vi "Teleop.vi"(10 "Match Info":T1={"Autonomous Elapsed Seconds"=0.0, "TeleOp Elapsed Seconds"=0.0, "Disabled Elapsed Seconds"=0.0, "Visited Autonomous"=FALSE, "Visited TeleOp"=FALSE, "Visited Disabled"=FALSE, "Autonomous Settings"={"Autonomous Style"=enum."Independent", "VI Refnum"=refnum}}, 11 "Call Context":T2) -> ()   [LabVIEW 2015]
doc: "This VI is called for each TeleOp packet received from the DS where the robot is not disabled. It is often used to read from the joysticks and update I/O or to update setpoints for timed control loops. It should complete and return within 20 milliseconds or it may miss DS packets."
uses:
  <vilib>/Rock Robotics/WPI/DriverStation/WPI_DriverStationDerivedRobotMode.ctl
  <vilib>/Rock Robotics/WPI/DriverStation/WPI_DriverStationMatch Info.ctl
  <vilib>/Rock Robotics/Network Tables/NT Read Boolean.vi
  <vilib>/Rock Robotics/Network Tables/NT Read Number.vi
  Robot Global Data.vi
panel:
  out "Sample Slider 0":dbl(slide) scale=0.0..5.0
  out "Sample Boolean 1":bool
  out "Sample Boolean 0":bool
  # "TELEOP.VI"
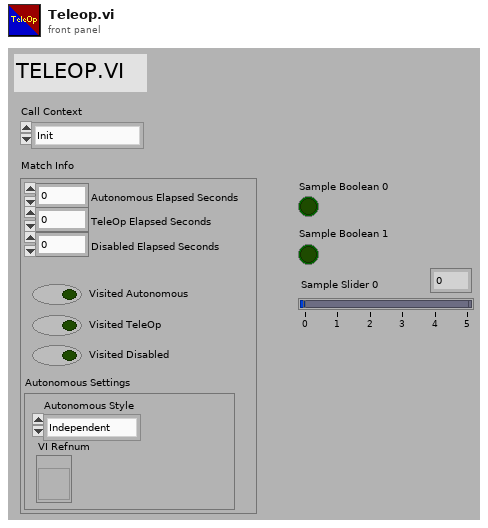
[diagram p1: front panel]
types:
  T1 = typedef "WPI_DriverStationMatch Info.ctl" = cluster{"Autonomous Elapsed Seconds":dbl, "TeleOp Elapsed Seconds":dbl, "Disabled Elapsed Seconds":dbl, "Visited Autonomous":bool, "Visited TeleOp":bool, "Visited Disabled":bool, "Autonomous Settings":cluster{"Autonomous Style":enum16{"Iterative", "Independent"}, "VI Refnum":refnum<vi>}}
  T2 = typedef "WPI_DriverStationDerivedRobotMode.ctl" = enum16{"Init", "Execute", "Stop"}
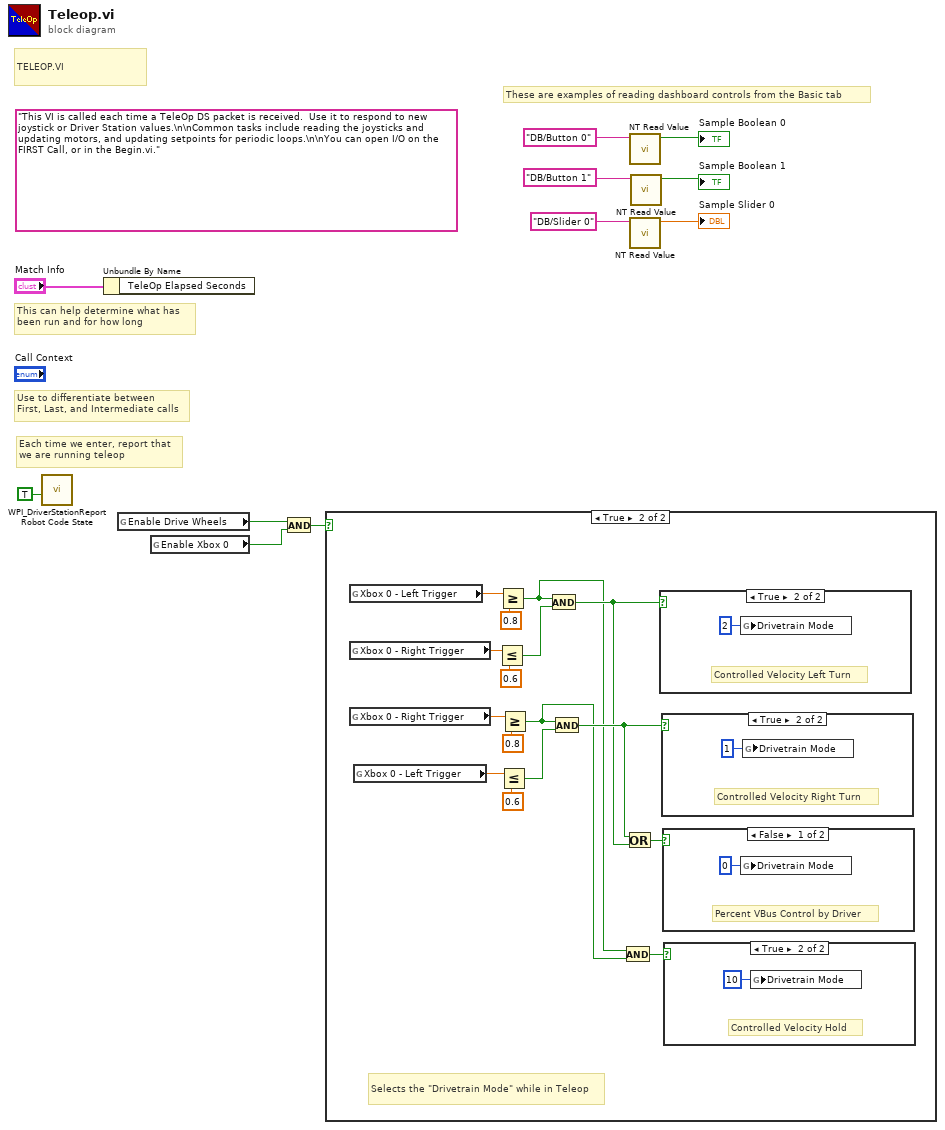
[diagram p0: block diagram]
diagram:
  (unwired) "This VI is called each time a TeleOp DS packet is received.  Use it to respond to new joystick or Driver Station values.\n\nCommon tasks include reading the joysticks and updating motors, and updating setpoints for periodic loops.\n\nYou can open I/O on the FIRST Call, or in the Begin.vi."
  # "TELEOP.VI"
  # "These are examples of reading dashboard controls from the Basic tab"
  # "Each time we enter, report that\nwe are running teleop"
  # "Use to differentiate between\nFirst, Last, and Intermediate calls"
  # "This can help determine what has\nbeen run and for how long"
  n1 = call <vilib>:"WPI_DriverStationReport Robot Code State.vi"("TeleOp"=TRUE ("Autonomous")) -> ()  [unwired: 10 in, 1 out]
  n2 = Unbundle By Name("Match Info") -> ()  [unwired: 1 out]
  n3 = global read "Robot Global Data.vi" "Enable Drive Wheels"() -> (w2:bool)
  n4 = global read "Robot Global Data.vi" "Enable Xbox 0"() -> (w1:bool)
  n5 = And(x=w2, y=w1) -> (x .and. y?=w3:bool)
  n6 = case shown="True" w3 {
    frame False {
    }
    frame True {
      # "Selects the \"Drivetrain Mode\" while in Teleop"
      n7 = global read "Robot Global Data.vi" "Xbox 0 - Left Trigger"() -> (w27:dbl)
      n8 = global read "Robot Global Data.vi" "Xbox 0 - Right Trigger"() -> (w25:dbl)
      n9 = global read "Robot Global Data.vi" "Xbox 0 - Right Trigger"() -> (w22:dbl)
      n10 = global read "Robot Global Data.vi" "Xbox 0 - Left Trigger"() -> (w20:dbl)
      n11 = Less Or Equal?(x=w25, y=0.6) -> (x <= y?=w23:bool)
      n12 = Greater Or Equal?(x=w27, y=0.8) -> (x >= y?=w14:bool)
      n13 = Less Or Equal?(x=w20, y=0.6) -> (x <= y?=w18:bool)
      n14 = Greater Or Equal?(x=w22, y=0.8) -> (x >= y?=w13:bool)
      n15 = And(x=w14, y=w23) -> (x .and. y?=w15:bool)
      n16 = And(x=w13, y=w18) -> (x .and. y?=w16:bool)
      n17 = And(x=w14, y=w13) -> (x .and. y?=w12:bool)
      n18 = Or(x=w16, y=w15) -> (x .or. y?=w17:bool)
      n19 = case shown="True" w15 {
        frame False {
        }
        frame True {
          # "Controlled Velocity Left Turn"
          n20 = global write "Robot Global Data.vi" "Drivetrain Mode"(u16 2 ("Drivetrain Mode")) -> ()
        }
      }
      n21 = case shown="True" w16 {
        frame False {
        }
        frame True {
          # "Controlled Velocity Right Turn"
          n22 = global write "Robot Global Data.vi" "Drivetrain Mode"(u16 1 ("Drivetrain Mode")) -> ()
        }
      }
      n23 = case shown="False" w17 {
        frame False {
          # "Percent VBus Control by Driver"
          n24 = global write "Robot Global Data.vi" "Drivetrain Mode"(u16 0 ("Drivetrain Mode")) -> ()
        }
        frame True {
        }
      }
      n25 = case shown="True" w12 {
        frame False {
        }
        frame True {
          # "Controlled Velocity Hold"
          n26 = global write "Robot Global Data.vi" "Drivetrain Mode"(u16 10 ("Drivetrain Mode")) -> ()
        }
      }
    }
  }
  n27 = call-poly <vilib>:"NT Read Value.vi"("Name"="DB/Button 0" ("refnum name")) -> ("Boolean"=→"Sample Boolean 0":bool)  [unwired: 9 in, 1 out]
  n28 = call-poly <vilib>:"NT Read Value.vi"("Name"="DB/Slider 0" ("refnum name")) -> ("Numeric"=→"Sample Slider 0":dbl)  [unwired: 9 in, 1 out]
  n29 = call-poly <vilib>:"NT Read Value.vi"("Name"="DB/Button 1" ("refnum name")) -> ("Boolean"=→"Sample Boolean 1":bool)  [unwired: 9 in, 1 out]
